vi "Timed Task.vi"(9 "Time (ms)":i32, 11 "Start":bool=TRUE) -> (3 "Running":bool)   [LabVIEW 2014]
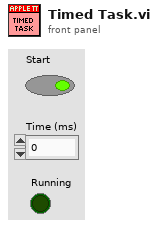
[diagram p1: front panel]
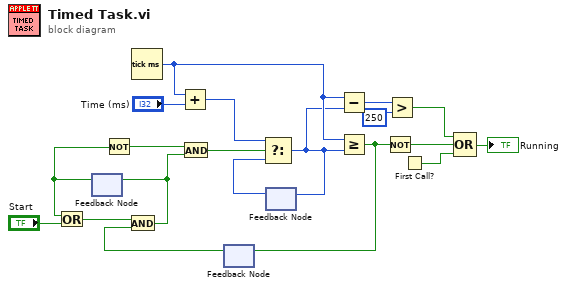
[diagram p0: block diagram]
diagram:
  n1 = feedback #1() -> (w13:bool)  [unwired: 1 in]
  n2 = Or(x=w13, y="Start") -> (x .or. y?=w15:bool)
  n3 = Not(x=w13) -> (.not. x?=w12:bool)
  n4 = Tick Count (ms)() -> (millisecond timer value=w2:u32)
  n5 = Add(x=w2, y="Time (ms)") -> (x+y=w18:u32)
  n6 = feedback #2() -> (w9:bool)  [unwired: 1 in]
  n7 = And(x=w15, y=w9) -> (x .and. y?=w11:bool)
  n8 = feedback-in #1(w11) -> ()
  n9 = And(x=w12, y=w11) -> (x .and. y?=w16:bool)
  n10 = feedback #3() -> (w17:u32)  [unwired: 1 in]
  n11 = Select(t=w18, s=w16, f=w17) -> (s? t:f=w1:u32)
  n12 = feedback-in #3(w1) -> ()
  n13 = Subtract(x=w2, y=w1) -> (x-y=w4:u32)
  n14 = Greater Or Equal?(x=w2, y=w1) -> (x >= y?=w10:bool)
  n15 = feedback-in #2(w10) -> ()
  n16 = Not(x=w10) -> (.not. x?=w7:bool)
  n17 = Greater?(x=w4, y=u32 250) -> (0:w3:bool)
  n18 = First Call?() -> (First Call?: T/F=w6:bool)
  n19 = Compound Arithmetic op=OR(w3, w7, w6) -> (→"Running":bool)
